vi "5.1 EMGtoOMG OFFLINE.vi"() -> ()   [LabVIEW 2018]
panel:
  in  "s 3":bool
  in  "s 2":bool
  in  "s":bool
  out "?":bool
  out "?":bool
  out "?":bool
  out "?":bool
  out "?":bool
  out "?":bool
  out "?":bool
  out "?":bool
  out "?":bool
  in  "file path (use dialog) 2":path
  in  "rate":dbl=5000.0
  in  "sample size":i32=5000
  out "return value":string
  out "charSearch":dbl[](array[numeric])
  out "setID":dbl[](array[numeric])
  in  "stop":bool
  in  "module path":path
  # "1-1-3     3 (x8) \"G\"     1-2-1     3 (x4) \"o\"     2\n\n1-1-2     3 (x2) \"b\"     1-2-1     3 (x1) \"l\"     1-2-2     3 (x5) \"u\"     1-1-2     3 (x5) \"e\"     2\n\n1-3-1     3 (x4) \"!\"     1-1-1     2     3 (x2)     2     1"
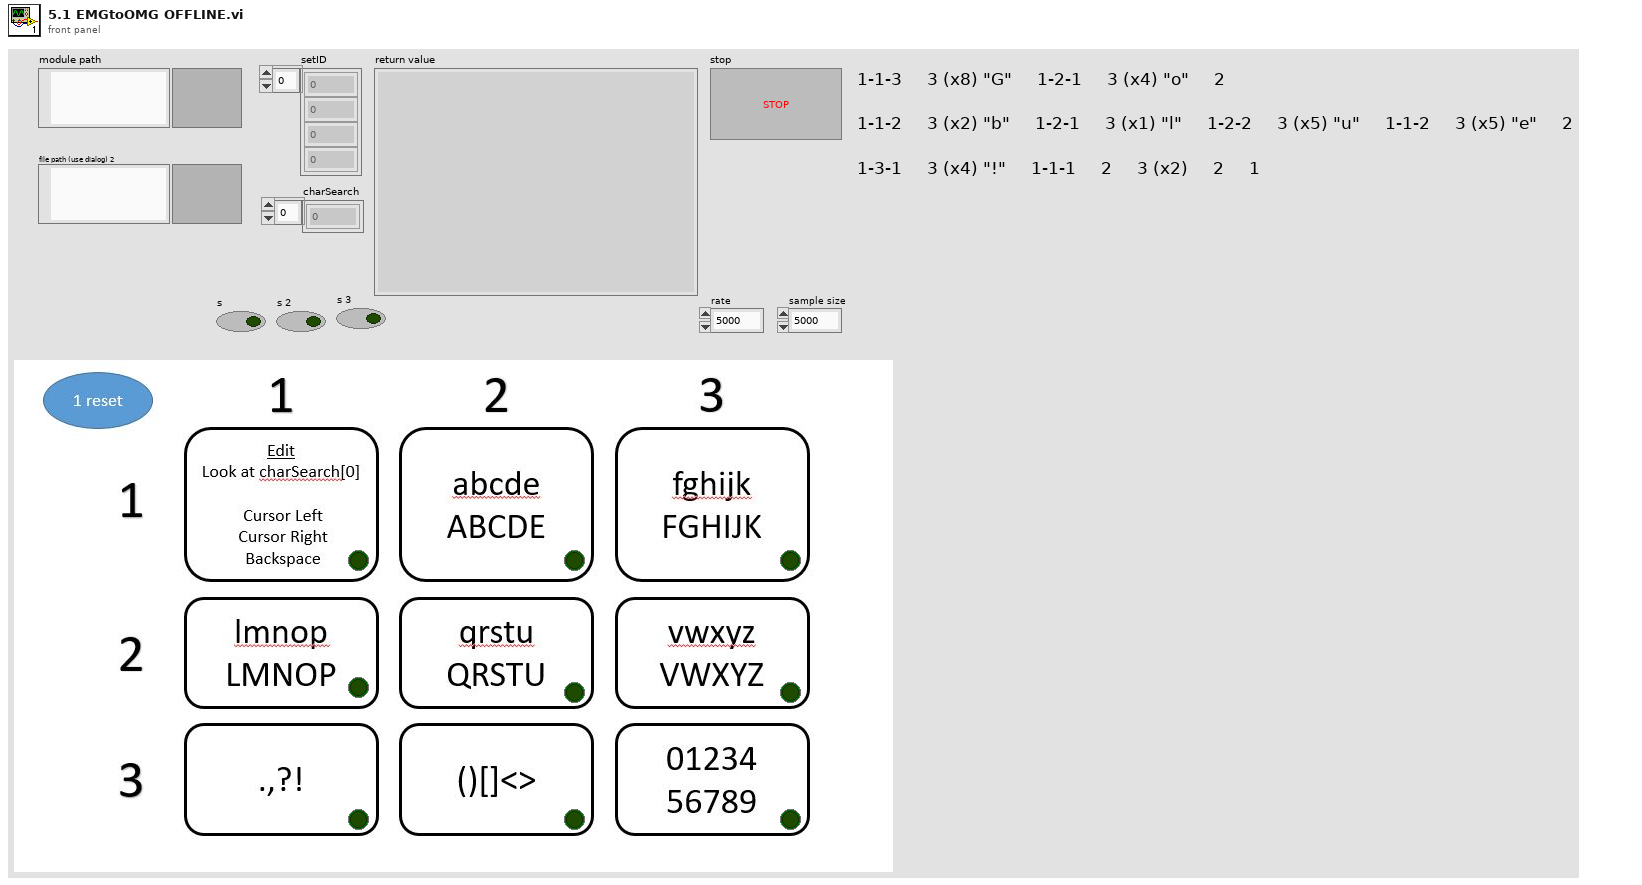
[diagram p1: front panel]
types:
  T1 = enum16{"open", "replace", "create", "open or create", "replace or create", "replace or create with confirmation"}
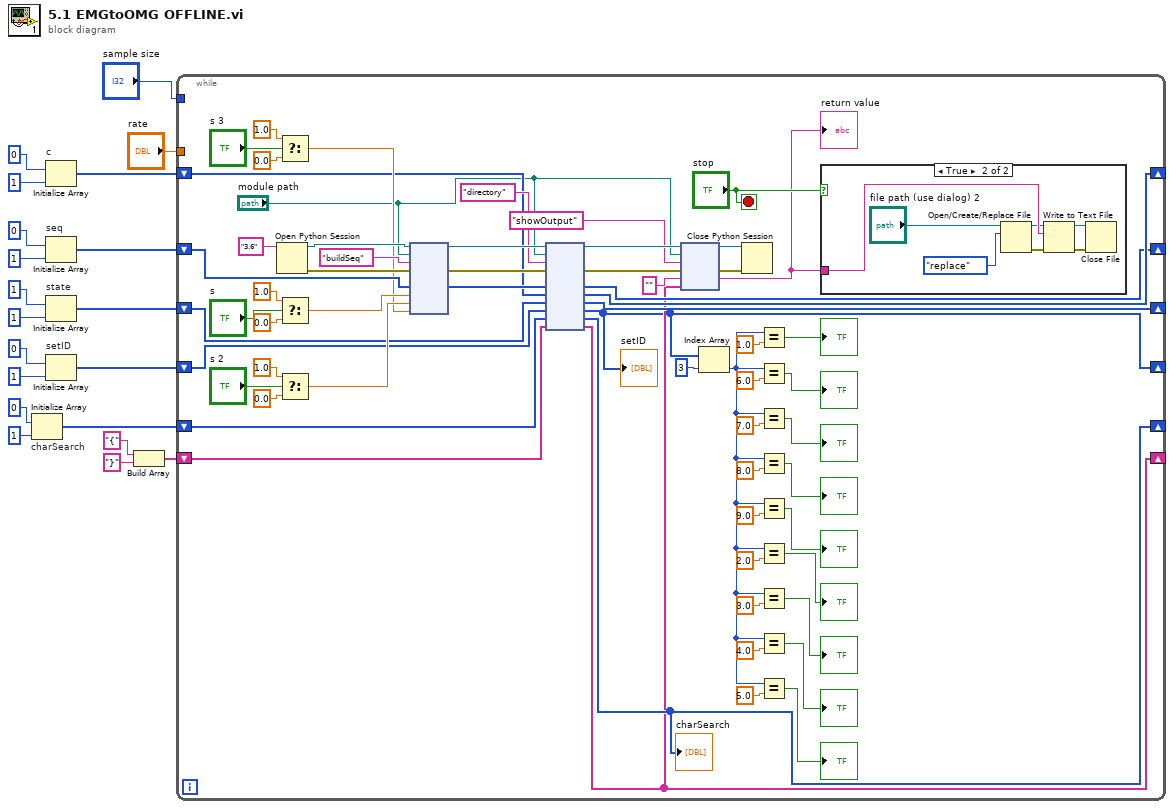
[diagram p0: block diagram]
diagram:
  n1 = Initialize Array "charSearch"(0, 1 ("dimension size")) -> (w15:i32[])
  n2 = Initialize Array "c"(0, 1 ("dimension size")) -> (w13:i32[])
  n3 = Initialize Array "seq"(0, 1 ("dimension size")) -> (w20:i32[])
  n4 = Initialize Array "state"(1, 1 ("dimension size")) -> (w10:i32[])
  n5 = Initialize Array "setID"(0, 1 ("dimension size")) -> (w16:i32[])
  n6 = Build Array("{", "}") -> (w7:string[])
  n7 = while {
    shift-right: [w46] -> _
    shift-left: w20 -> [w74]
    shift-right: [w44] -> _
    shift-left: w16 -> [w63]
    shift-right: [w49] -> _
    shift-left: w15 -> [w62]
    shift-right: [w45] -> _
    shift-left: w7 -> [w61]
    shift-right: [w59] -> _
    shift-left: w10 -> [w60]
    shift-right: [w57] -> _
    shift-left: w13 -> [w58]
    tunnel: "sample size" -> [_]
    tunnel: "rate" -> [_]
    stop <- "stop" stop-if-true
    n8 = Open Python Session(python version="3.6" ("Python version")) -> (session out=w80:refnum<k35>, error out=w79:errorcluster)  [unwired: 2 in]
    n9 = Select(t=1.0, s="s 3", f=0.0) -> (s? t:f=w68:dbl)
    n10 = Select(t=1.0, s="s", f=0.0) -> (s? t:f=w77:dbl)
    n11 = Select(t=1.0, s="s 2", f=0.0) -> (s? t:f=w69:dbl)
    n12 = node(w80, "module path", "buildSeq" ("function name"), w79, w74, w77, w69, w68) -> (w67:refnum<k35>, w66:errorcluster, w64:i32[])  [unwired: 5 in, 2 out]
    n13 = node(w67, "module path", "directory" ("function name"), w66, w64, w58, w60, w63, w62, w61) -> (w55:refnum<k35>, w53:errorcluster, w46:i32[], w57:i32[], w59:i32[], w44:i32[], w49:i32[], w45:string[])  [unwired: 2 in, 2 out]
    "setID" <- w44
    "charSearch" <- w49
    n14 = node(w55, "module path", "showOutput" ("function name"), w53, "", w45) -> (w54:refnum<k35>, w52:errorcluster, w47:string)  [unwired: 1 in, 2 out]
    "return value" <- w47
    n15 = Index Array(array=w44, index=3) -> (element=w24:i32)
    n16 = Close Python Session(session in=w54, error in=w52) -> ()  [unwired: 1 out]
    n17 = Equal?(x=w24, y=1.0) -> (x = y?=→"?":bool)
    n18 = Equal?(x=w24, y=6.0) -> (x = y?=→"?":bool)
    n19 = Equal?(x=w24, y=7.0) -> (x = y?=→"?":bool)
    n20 = Equal?(x=w24, y=8.0) -> (x = y?=→"?":bool)
    n21 = Equal?(x=w24, y=9.0) -> (x = y?=→"?":bool)
    n22 = Equal?(x=w24, y=2.0) -> (x = y?=→"?":bool)
    n23 = Equal?(x=w24, y=3.0) -> (x = y?=→"?":bool)
    n24 = Equal?(x=w24, y=4.0) -> (x = y?=→"?":bool)
    n25 = Equal?(x=w24, y=5.0) -> (x = y?=→"?":bool)
    n26 = case shown="True" "stop" {
      tunnel: w47 -> [_ w88]
      frame False {
      }
      frame True {
        n27 = Open/Create/Replace File(file path (use dialog)="file path (use dialog) 2", operation (0:open)=T1."replace") -> (refnum out=w84:refnum<file>, error out=w85:errorcluster)  [unwired: 4 in, 1 out]
        n28 = Write to Text File(file (use dialog)=w84, text=w88, error in=w85) -> (refnum out=w86:refnum<file>, error out=w87:errorcluster)  [unwired: 1 in, 1 out]
        n29 = Close File(refnum=w86, error in=w87) -> ()  [unwired: 2 out]
      }
    }
  }
